vi "Grava_EQ_u.vi"(3 "all Layers EQ_DATA+REPORT":u32[](array[numeric]) format="%x", 4 "number of pixels":u32, 5 "Folder path: equalization":path) -> (1 "subfolder path: text reports":path)   [LabVIEW 2015, in "VIPM2.lvlib"]
uses:
  VIPM2.lvlib
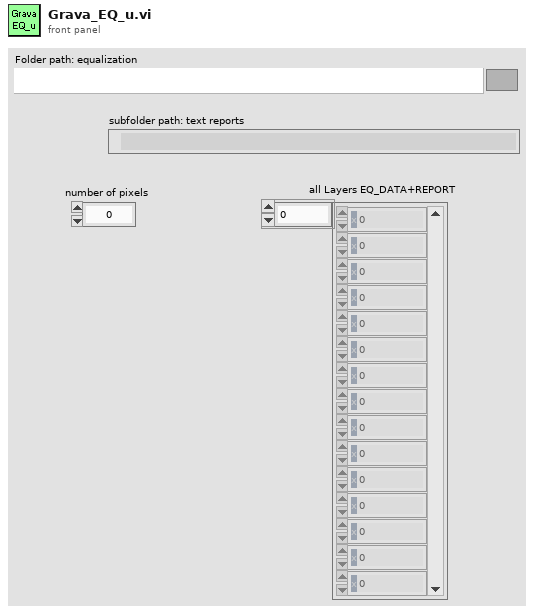
[diagram p1: front panel]
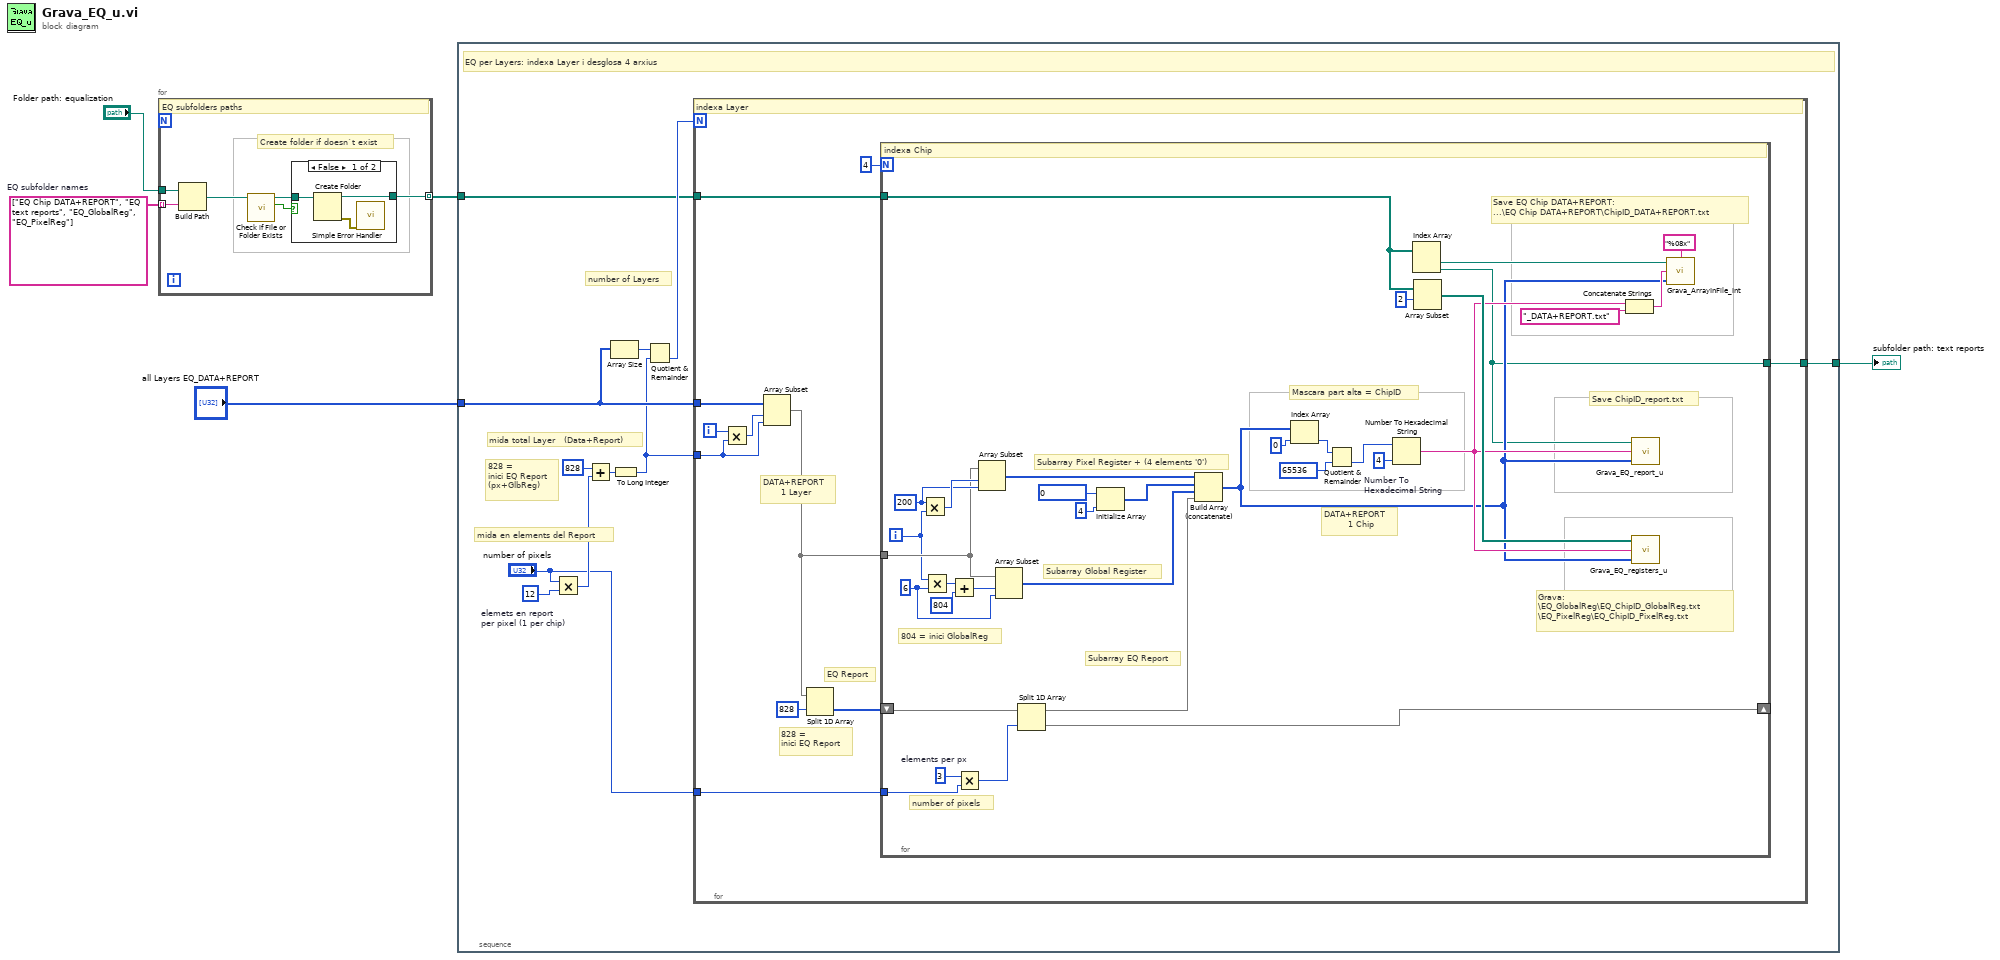
[diagram p0: block diagram]
diagram:
  w3 = string[] ["EQ Chip DATA+REPORT", "EQ text reports", "EQ_GlobalReg", "EQ_PixelReg"]  # EQ subfolder names
  n1 = for {
    tunnel: w3 -> [w8] mode=indexing
    tunnel: "Folder path: equalization" -> [w7]
    tunnel: [w6] -> w2 mode=indexing
    # "Create folder if doesn`t exist"
    # "EQ subfolders paths"
    n2 = Build Path(base path=w7, name or relative path=w8) -> (appended path=w9:path)
    n3 = call <vilib>:"Check if File or Folder Exists.vi"("path"=w9) -> ("file or folder exists?"=w11:bool, "dup path"=w10:path)  [unwired: 8 in, 1 out]
    n4 = case shown="False" w11 {
      tunnel: w10 -> [w14 w15]
      tunnel: [w13 w15] -> w6
      frame False {
        n5 = Create Folder(path (use dialog)=w14) -> (created path=w13:path, error out=w12:errorcluster)  [unwired: 2 in, 1 out]
        n6 = call <vilib>:"Simple Error Handler.vi"("error in (no error)"=w12) -> ()  [unwired: 4 in, 5 out]
      }
      frame True {
      }
    }
  }
  n7 = stacked-sequence {
    tunnel: "all Layers EQ_DATA+REPORT" -> [w22]
    tunnel: w2 -> [w17]
    tunnel: [w16] -> w1
    frame #0 {
      w26 = u32 12  # elemets en report per pixel (1 per chip)
      # "number of Layers"
      # "mida total Layer   (Data+Report)"
      # "828 =\ninici EQ Report\n(px+GlbReg)"
      # "mida en elements del Report"
      # "EQ per Layers: indexa Layer i desglosa 4 arxius"
      n8 = Multiply(x="number of pixels", y=w26) -> (x*y=w24:u32)
      n9 = Add(x=u32 828, y=w24) -> (x+y=w19:u32)
      n10 = Array Size(array=w22) -> (size(s)=w21:i32)
      n11 = To Long Integer(number=w19) -> (32bit integer=w18:i32)
      n12 = Quotient & Remainder(x=w21, y=w18) -> (floor(x/y)=w20:i32)  [unwired: 1 out]
      n13 = for {
        N: w20 -> [_]
        tunnel: w22 -> [w33]
        tunnel: "number of pixels" -> [w34]
        tunnel: w18 -> [w31]
        tunnel: w17 -> [w28]
        tunnel: [w27] -> w16
        i -> [w29]
        # "DATA+REPORT\n      1 Layer"
        # "EQ Report"
        # "828 =\ninici EQ Report"
        # "indexa Layer"
        n14 = Multiply(x=w29, y=w31) -> (x*y=w32:i32)
        n15 = Array Subset "Array Subset"(array=w33, index=w32, length=w31) -> (w30:u32[])
        n16 = Split 1D Array(array=w30, index=828) -> (second subarray=w35:u32[])  [unwired: 1 out]
        n17 = for {
          N: 4 -> [_]
          tunnel: w30 -> [w65]
          shift-right: [w57] -> _
          shift-left: w35 -> [w59]
          tunnel: w34 -> [w52]
          tunnel: w28 -> [w44]
          tunnel: [w39] -> w27
          i -> [w53]
          w51 = u32 3  # elements per px
          w66 = 6 ("length")
          w70 = 200 ("length")
          # "Save ChipID_report.txt"
          # "Save EQ Chip DATA+REPORT:\n...\\EQ Chip DATA+REPORT\\ChipID_DATA+REPORT.txt"
          # "DATA+REPORT\n        1 Chip"
          # "Grava:\n\\EQ_GlobalReg\\EQ_ChipID_GlobalReg.txt\n\\EQ_PixelReg\\EQ_ChipID_PixelReg.txt"
          # "number of pixels"
          # "Mascara part alta = ChipID"
          # "Subarray EQ Report"
          # "Subarray Global Register"
          # "Subarray Pixel Register + (4 elements '0')"
          # "804 = inici GlobalReg"
          # "indexa Chip"
          n18 = Multiply(x=w70, y=w53) -> (x*y=w71:i32)
          n19 = Multiply(x=w53, y=w66) -> (x*y=w69:i32)
          n20 = Add(x=w69, y=804) -> (x+y=w67:i32)
          n21 = Multiply(x=w51, y=w52) -> (x*y=w50:u32)
          n22 = Array Subset "Array Subset"(array=w65, index=w71, length=w70) -> (w63:u32[])
          n23 = Array Subset(array=w65, index=w67, length=w66) -> (w60:u32[])
          n24 = Split 1D Array(array=w59, index=w50) -> (first subarray=w58:u32[], second subarray=w57:u32[])
          n25 = Initialize Array(u32 0 ("dimension size"), 4 ("dimension size")) -> (w61:u32[])
          n26 = Build Array (concatenate)(w63, w61, w60, w58) -> (w40:u32[])
          n27 = Index Array "Index Array"(array=w40, index=0) -> (element=w54:u32)
          n28 = Quotient & Remainder(x=w54, y=u32 65536) -> (floor(x/y)=w48:u32)  [unwired: 1 out]
          n29 = Number To Hexadecimal String "Number To\nHexadecimal String"(1:i16 4 ("width (-)"), 2:w48) -> (0:w41:string)
          n30 = Index Array "Index Array"(array=w44) -> (element #1=w47:path, element #2=w39:path)  [unwired: 2 in]
          n31 = Array Subset "Array Subset"(array=w44, index=2) -> (w42:path[])  [unwired: 1 in]
          n32 = Concatenate Strings(w41, "_DATA+REPORT.txt" ("string")) -> (w46:string)
          n33 = call "Grava_EQ_report_u.vi"("EQ Data+Report_u (hex)"=w40, "ChipID (file name)"=w41, "EQ_u folder path"=w39) -> ()  [unwired: 1 in]
          n34 = call "Grava_EQ_registers_u.vi"("EQ Data+Report_u (hex)"=w40, "ChipID (file name)"=w41, "EQ_u file paths"=w42) -> ()  [unwired: 3 in]
          n35 = call "Grava_ArrayInFile_int.vi"("format (%08x)"="%08x", "Array to save"=w40, "file name"=w46, "folder path"=w47) -> ()  [unwired: 1 in]
        }
      }
    }
  }
  "subfolder path: text reports" <- w1
